vi "ADC_Read.vi"(0 "GPIB Address":T2=8, 5 "Ch & spans":T1[](array[typedef]) {"low limit (-10V)" format="%.3f"; "high limit (10V)" format="%.3f"}, 7 "number of scans to read":i32=1000, 11 "error in (no error)":errorcluster) -> (8 "binary data":i16[][](array[numeric]), 15 "error out":errorcluster)   [LabVIEW 2010]
doc: "This VI reads data from a buffered data acquisition.\n\nBefore reading any data, AI Read checks to see if the input cluster error in indicates that an error has already occurred. If so, this VI does not read any data, but passes the error information unmodified through error out. Otherwise, this VI calls the Analog Input Buffer Read VI to read the specified amount of data from a buffered analog input acquisition.\n\nInput Values:\n\n(u32) taskID in: identifies the group and I/O operation.\n\n(i32) number of scans to read: specifies the number of scans to retrieve from the acquisition buffer. The default input is -1 which tells LabVIEW to set number of scans to read equal to the value of the number of scans to acquire control when AI Start was called. If number of scans to read is -1 and number of scans to acquire was 0 then LabVIEW will set number of scans to read to 100.\n\n(sgl) time limit in sec: defines the timeout for the read operation. The VI will wait this long for the requested amount of data to be available before returning a timeout warning code. The default input is -1.0, which tells LabVIEW not to change the time limit setting. The default setting is 1 sec. The resolution of the timeout clock is about 55Êmsec.\n\n(u16) output units: specifies whether the VI returns unscaled binary data and/or scaled data.\n 0: Do not change the output type setting. \n 1: Return scaled data only (default input and setting). \n 2: Return binary data only. \n 3: Return scaled and binary data.\n\n(cluster) read position: defines where you want to read from the acquisition buffer with the following parameters:\n \n (u16) position: indicates which reference mark \n within an input buffer provides the reference point \n for the read.\n 0: Do not change (default input). \n 1: Relative to the read mark (default setting). \n 2: Relative to the start of buffer. \n 3: Relative to the end of data. \n 4: Relative to the trigger point\n (only valid when acquisition is complete).\n\n (i32) read offset: the VI adds read offset scans\n to the mark specified by position to determine\n the starting point for the read.\n\n(cluster) error in: a cluster describing any error conditions prior to this VI's execution. The default input of this cluster is no error. If an error has already occurred, this VI does not read any data, it just passes the values of taskID in and error in to taskID out and error out. The error in cluster contains the following parameters: \n\n (bool) status: TRUE if an error has occurred.\n If status is TRUE, this VI does not read any\n data.\n\n (i32) code: the error code associated with an error.\n A value of 0 means no error, a negative value is an error,\n and a positive value is a warning.\n\n (string) source: an indication of where an \n error occurred, usually the name of the VI.\n\nOutput Values:\n\n(u32) taskID out: the same as taskID in; identifies the group and I/O operation.\n\n([[sgl]]) scaled data: a two-dimensional array that contains scaled analog input data if output units requests scaled data. The first dimension is scans, the second dimension is channels.\n\n([[i16]]) binary data: a two-dimensional array that contains unscaled analog input data if output units requests binary data. The first dimension is scans, the second dimension is channels.\n\n(bool) retrieval complete: TRUE when the acquisition finishes and no backlog data remains to be read.\n\n(i32) number read: the number of scans returned. This will be the same as number of scans to read unless an error or timeout occurs or the VI reaches the end of the data.\n\n(i32) scan backlog: the amount of data acquired minus the amount of data read. If scan backlog increases each time you read data, you are not reading data fast enough to keep up with the acquisition, and you may get an overwrite error. Decrease your scan rate, increase the number of scans to read, read the scans more often, or increase the buffer size. See the description of the Analog Input Buffer Read VI for a precise definition of how scan backlog is computed.\n\n(cluster) error out: a cluster containing error information. If error in indicated an error, error out contains the same error information. Otherwise, it describes the error status of this VI. Use the General Error Handler utility VI to check the error at the end of your diagram. The error out cluster contains the following parameters: \n\n (bool) status: TRUE if an error has occurred.\n\n (i32) code: the error code associated with an error.\n A value of 0 means no error, a negative value is an error,\n and a positive value is a warning.\n\n (string) source: an indication of where an \n error occurred, usually the name of the VI."
uses:
  ADC_GPIB_address.ctl
  Controls/Ch_and_Spans.ctl
panel:
  # "channel"
  # "scan #"
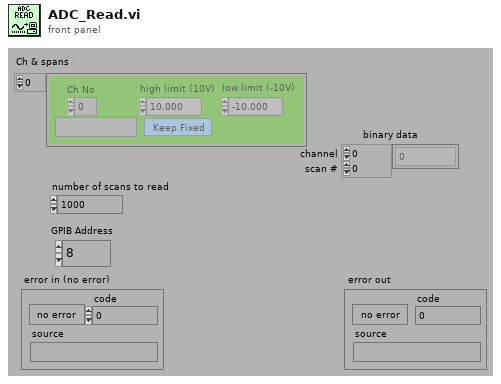
[diagram p1: front panel]
types:
  T1 = typedef "Ch_and_Spans.ctl" = cluster{"high limit (10V)":sgl, "low limit (-10V)":sgl, "Ch No":i16, "Var name":string, "Use Latest Calib":bool}
  T2 = typedef "ADC_GPIB_address.ctl" = u8
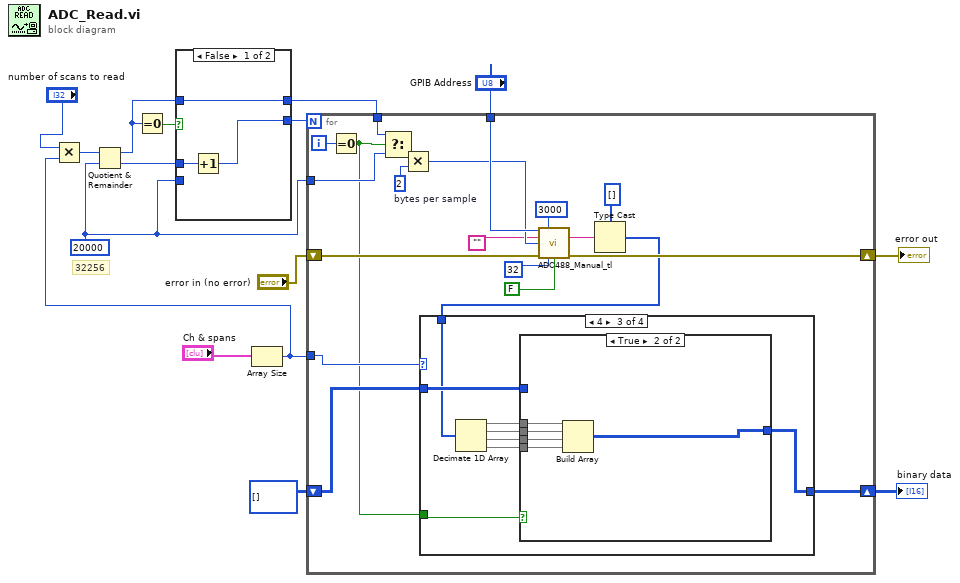
[diagram p0: block diagram]
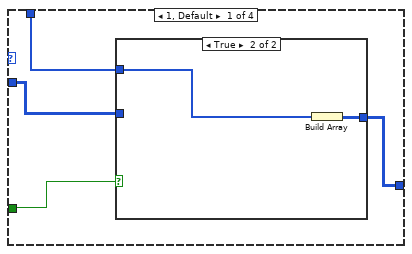
[diagram p3: hidden frame]
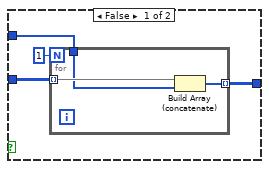
[diagram p4: hidden frame]
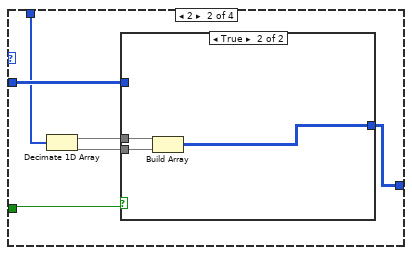
[diagram p5: hidden frame]
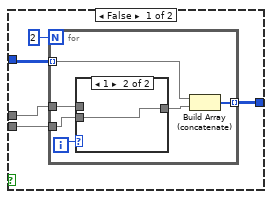
[diagram p6: hidden frame]
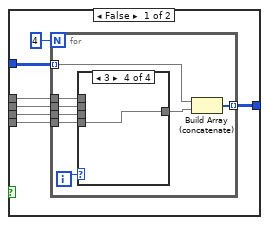
[diagram p8: hidden frame]
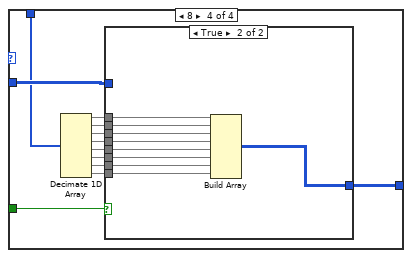
[diagram p12: hidden frame]
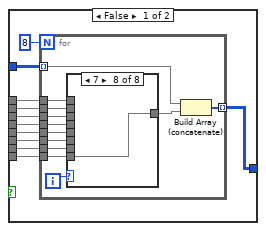
[diagram p13: hidden frame]
diagram:
  w5 = 20000 ("y")
  # "32256"
  n1 = Array Size(array="Ch & spans") -> (size(s)=w2:i32)
  n2 = Multiply(x="number of scans to read", y=w2) -> (x*y=w11:i32)
  n3 = Quotient & Remainder(x=w11, y=w5) -> (x-y*floor(x/y)=w3:i32, floor(x/y)=w6:i32)
  n4 = Equal To 0?(x=w3) -> (x = 0?=w8:bool)
  n5 = case shown="False" w8 {
    tunnel: [w16 w20] -> w7
    tunnel: w6 -> [w17 w20]
    tunnel: [w18 w19] -> w4
    tunnel: w5 -> [_ w19]
    tunnel: w3 -> [w18 _]
    frame False {
      n6 = Increment(x=w17) -> (x+1=w16:i32)
    }
    frame True {
    }
  }
  n7 = for {
    N: w7 -> [_]
    tunnel: "GPIB Address" -> [w38]
    shift-right: [w23] -> w9
    shift-left: i16[][] [] -> [w22]
    tunnel: w4 -> [w36]
    tunnel: w5 -> [w35]
    shift-right: [w32] -> w13
    shift-left: "error in (no error)" -> [w27]
    tunnel: w2 -> [w25]
    i -> [w37]
    w34 = 2  # bytes per sample
    n8 = Equal To 0?(x=w37) -> (x = 0?=w21:bool)
    n9 = Select(t=w36, s=w21, f=w35) -> (s? t:f=w26:i32)
    n10 = Multiply(x=w26, y=w34) -> (x*y=w33:i32)
    n11 = call "ADC488_Manual_tl.vi"("Clear device prior to command String"=FALSE, "Timeout in msec"=3000, "Serial Poll Byte"=u8 32, "GPIB Address"=w38, "Command String"="", "Byte Count Requested"=w33, "error in (no error)"=w27) -> ("Response String"=w40:string, "error out"=w32:errorcluster)  [unwired: 7 out]
    n12 = Type Cast(type=i16[] [], x=w40) -> (*(type *) &x=w24:i16[])
    n13 = case shown="4" w25 {
      tunnel: w24 -> [w43 w57 w81 w117]
      tunnel: w22 -> [w44 w59 w83 w119]
      tunnel: [w42 w58 w82 w118] -> w23
      tunnel: w21 -> [w41 w54 w76 w108]
      frame 1, Default {
        n14 = case shown="True" w41 {
          tunnel: w44 -> [w48 _]
          tunnel: w43 -> [w47 w53]
          tunnel: [w45 w52] -> w42
          frame False {
            n15 = for {
              N: 1 -> [_]
              tunnel: w48 -> [w51] mode=indexing
              tunnel: w47 -> [w50]
              tunnel: [w49] -> w45 mode=indexing
              n16 = Build Array (concatenate)(w51, w50) -> (w49:i16[])
            }
          }
          frame True {
            n17 = Build Array(w53) -> (w52:i16[][])
          }
        }
      }
      frame 2 {
        n18 = Decimate 1D Array(w57) -> (w56:i16[], w55:i16[])
        n19 = case shown="True" w54 {
          tunnel: w59 -> [w64 _]
          tunnel: [w63 w73] -> w58
          tunnel: w56 -> [w62 w75]
          tunnel: w55 -> [w60 w74]
          frame False {
            n20 = for {
              N: 2 -> [_]
              tunnel: w64 -> [w70] mode=indexing
              tunnel: [w69] -> w63 mode=indexing
              tunnel: w62 -> [w66]
              tunnel: w60 -> [w65]
              i -> [w68]
              n21 = case shown="1" w68 {
                tunnel: [w71 w72] -> w67
                tunnel: w66 -> [w71 _]
                tunnel: w65 -> [_ w72]
                frame 0, Default {
                }
                frame 1 {
                }
              }
              n22 = Build Array (concatenate)(w70, w67) -> (w69:i16[])
            }
          }
          frame True {
            n23 = Build Array(w75, w74) -> (w73:i16[][])
          }
        }
      }
      frame 4 {
        n24 = Decimate 1D Array(w81) -> (w79:i16[], w80:i16[], w78:i16[], w77:i16[])
        n25 = case shown="True" w76 {
          tunnel: w83 -> [w90 _]
          tunnel: [w89 w103] -> w82
          tunnel: w80 -> [w87 w106]
          tunnel: w79 -> [w86 w107]
          tunnel: w78 -> [w85 w105]
          tunnel: w77 -> [w84 w104]
          frame False {
            n26 = for {
              N: 4 -> [_]
              tunnel: w90 -> [w98] mode=indexing
              tunnel: [w97] -> w89 mode=indexing
              tunnel: w87 -> [w94]
              tunnel: w86 -> [w93]
              tunnel: w85 -> [w92]
              tunnel: w84 -> [w91]
              i -> [w96]
              n27 = case shown="3" w96 {
                tunnel: [w99 w100 w101 w102] -> w95
                tunnel: w94 -> [_ w100 _ _]
                tunnel: w93 -> [w99 _ _ _]
                tunnel: w92 -> [_ _ w101 _]
                tunnel: w91 -> [_ _ _ w102]
                frame 0, Default {
                }
                frame 1 {
                }
                frame 2 {
                }
                frame 3 {
                }
              }
              n28 = Build Array (concatenate)(w98, w95) -> (w97:i16[])
            }
          }
          frame True {
            n29 = Build Array(w107, w106, w105, w104) -> (w103:i16[][])
          }
        }
      }
      frame 8 {
        n30 = Decimate 1D Array(w117) -> (w115:i16[], w116:i16[], w114:i16[], w113:i16[], w112:i16[], w111:i16[], w110:i16[], w109:i16[])
        n31 = case shown="True" w108 {
          tunnel: w119 -> [w130 _]
          tunnel: [w129 w151] -> w118
          tunnel: w116 -> [w127 w158]
          tunnel: w115 -> [w126 w159]
          tunnel: w114 -> [w125 w157]
          tunnel: w113 -> [w124 w156]
          tunnel: w112 -> [w123 w155]
          tunnel: w111 -> [w122 w154]
          tunnel: w110 -> [w121 w153]
          tunnel: w109 -> [w120 w152]
          frame False {
            n32 = for {
              N: 8 -> [_]
              tunnel: w130 -> [w142] mode=indexing
              tunnel: [w141] -> w129 mode=indexing
              tunnel: w127 -> [w138]
              tunnel: w126 -> [w137]
              tunnel: w125 -> [w136]
              tunnel: w124 -> [w135]
              tunnel: w123 -> [w134]
              tunnel: w122 -> [w133]
              tunnel: w121 -> [w132]
              tunnel: w120 -> [w131]
              i -> [w140]
              n33 = case shown="7" w140 {
                tunnel: [w143 w144 w145 w146 w147 w148 w149 w150] -> w139
                tunnel: w138 -> [_ w144 _ _ _ _ _ _]
                tunnel: w137 -> [w143 _ _ _ _ _ _ _]
                tunnel: w136 -> [_ _ w145 _ _ _ _ _]
                tunnel: w135 -> [_ _ _ w146 _ _ _ _]
                tunnel: w134 -> [_ _ _ _ w147 _ _ _]
                tunnel: w133 -> [_ _ _ _ _ w148 _ _]
                tunnel: w132 -> [_ _ _ _ _ _ w149 _]
                tunnel: w131 -> [_ _ _ _ _ _ _ w150]
                frame 0, Default {
                }
                frame 1 {
                }
                frame 2 {
                }
                frame 3 {
                }
                frame 4 {
                }
                frame 5 {
                }
                frame 6 {
                }
                frame 7 {
                }
              }
              n34 = Build Array (concatenate)(w142, w139) -> (w141:i16[])
            }
          }
          frame True {
            n35 = Build Array(w159, w158, w157, w156, w155, w154, w153, w152) -> (w151:i16[][])
          }
        }
      }
    }
  }
  "error out" <- w13
  "binary data" <- w9
